vi "sgp4Init.vi"(1 "satrec":T2) -> (0 "satrec 2":T1)   [LabVIEW 2015]
uses:
  <vilib>/imath/engines/lvmath/Plug In/_Char/NIMS_CH_character datatype.ctl
  <vilib>/imath/engines/lvmath2/RunTimeEngine/Managers/WorkSpace/UID Generator.vi
  <vilib>/imath/engines/lvmath2/RunTimeEngine/RunTimeType/NIMS_RunTimeType_From StrictType (excl LVString).vi
  <instcachedir>/0/NIMS_RunTimeType_From StrictType (excl LVString)_EB1C38A9BC5048DA9ABDA8F781E54D21.lvgen/NIMS_RunTimeType_From StrictType (excl LVString)_EB1C38A9BC5048DA9ABDA8F781E54D21_032.vi
  <instcachedir>/0/NIMS_RunTimeType_From StrictType (excl LVString)_EB1C38A9BC5048DA9ABDA8F781E54D21.lvgen/NIMS_RunTimeType_From StrictType (excl LVString)_EB1C38A9BC5048DA9ABDA8F781E54D21_030.vi
  <vilib>/imath/engines/lvmath/Plug In/_Char/NIMS_CH_String CV to Character 2D.vi
  <instcachedir>/0/NIMS_CH_String CV to Character 2D_EC8CCB3F0D074D66A728E5B1D55F815A.lvgen/NIMS_CH_String CV to Character 2D_EC8CCB3F0D074D66A728E5B1D55F815A_000.vi
  <instcachedir>/0/NIMS_RunTimeType_From StrictType (excl LVString)_EB1C38A9BC5048DA9ABDA8F781E54D21.lvgen/NIMS_RunTimeType_From StrictType (excl LVString)_EB1C38A9BC5048DA9ABDA8F781E54D21_001.vi
  <instcachedir>/0/NIMS_RunTimeType_From StrictType (excl LVString)_EB1C38A9BC5048DA9ABDA8F781E54D21.lvgen/NIMS_RunTimeType_From StrictType (excl LVString)_EB1C38A9BC5048DA9ABDA8F781E54D21_031.vi
  <vilib>/imath/engines/lvmath2/RunTimeEngine/Struct/NIMS_StructSetField.vi
  <vilib>/imath/engines/lvmath2/RunTimeEngine/Struct/NIMS_StructGetField.vi
  <vilib>/imath/engines/lvmath2/RunTimeEngine/RunTimeType/NIMS_RunTimeType_To Numeric.vi
  <instcachedir>/0/NIMS_RunTimeType_To Numeric_B134FEC7BFC54ED5998F4CFD2EE98288.lvgen/NIMS_RunTimeType_To Numeric_B134FEC7BFC54ED5998F4CFD2EE98288_007.vi
  <instcachedir>/0/NIMS_RunTimeType_To Numeric_B134FEC7BFC54ED5998F4CFD2EE98288.lvgen/NIMS_RunTimeType_To Numeric_B134FEC7BFC54ED5998F4CFD2EE98288_009.vi
  <instcachedir>/0/NIMS_RunTimeType_From StrictType (excl LVString)_EB1C38A9BC5048DA9ABDA8F781E54D21.lvgen/NIMS_RunTimeType_From StrictType (excl LVString)_EB1C38A9BC5048DA9ABDA8F781E54D21_000.vi
  <vilib>/imath/engines/lvmath2/RunTimeEngine/LocalVariableDefStatement/MC_LocalVariableDefStatement_Display.vi
  <instcachedir>/0/NIMS_RunTimeType_To Numeric_B134FEC7BFC54ED5998F4CFD2EE98288.lvgen/NIMS_RunTimeType_To Numeric_B134FEC7BFC54ED5998F4CFD2EE98288_008.vi
  <vilib>/imath/engines/lvmath2/RunTimeEngine/BuiltInFunctions/cos/NIMS_cos(C).vi
  <instcachedir>/0/NIMS_cos(C)_840A8FDA839D4E2AADB43697F53F61ED.lvgen/NIMS_cos(C)_840A8FDA839D4E2AADB43697F53F61ED_001.vi
  <vilib>/imath/engines/lvmath2/RunTimeEngine/ArithmeticOperatorToken/NIMS_ArithmeticOperator_power(S).vi
  <instcachedir>/0/NIMS_ArithmeticOperator_power(S)_DFB67823F1414E5097C86E39787D8CA8.lvgen/NIMS_ArithmeticOperator_power(S)_DFB67823F1414E5097C86E39787D8CA8_009.vi
  <vilib>/imathl/engines/lvmath/Functions/Error Handling/Create Error.vi
  <vilib>/imath/engines/lvmath2/RunTimeEngine/BuiltInFunctions/sin/NIMS_sin(C).vi
  <instcachedir>/0/NIMS_sin(C)_93B37CF23FEA46B381CCAA607B2209DC.lvgen/NIMS_sin(C)_93B37CF23FEA46B381CCAA607B2209DC_001.vi
  <vilib>/imath/engines/lvmath2/RunTimeEngine/BuiltInFunctions/rem/NIMS_rem_no checks.vi
  <instcachedir>/0/NIMS_rem_no checks_948DC4F3B45040069021B8F54D02F312.lvgen/NIMS_rem_no checks_948DC4F3B45040069021B8F54D02F312_000.vi
  <vilib>/imath/engines/lvmath2/RunTimeEngine/BuiltInFunctions/abs/NIMS_abs(signed).vi
  <instcachedir>/0/NIMS_abs(signed)_C4FCB8E6058B49B797C7C8D53CA5F6EC.lvgen/NIMS_abs(signed)_C4FCB8E6058B49B797C7C8D53CA5F6EC_002.vi
  <instcachedir>/0/NIMS_ArithmeticOperator_power(S)_DFB67823F1414E5097C86E39787D8CA8.lvgen/NIMS_ArithmeticOperator_power(S)_DFB67823F1414E5097C86E39787D8CA8_014.vi
  <instcachedir>/0/NIMS_ArithmeticOperator_power(S)_DFB67823F1414E5097C86E39787D8CA8.lvgen/NIMS_ArithmeticOperator_power(S)_DFB67823F1414E5097C86E39787D8CA8_010.vi
  <vilib>/imath/engines/lvmath2/RunTimeEngine/BuiltInFunctions/atan2/NIMS_atan2.vi
  <instcachedir>/0/NIMS_atan2_A91AA4A7D42247EDBE8F76DB99AF04A4.lvgen/NIMS_atan2_A91AA4A7D42247EDBE8F76DB99AF04A4_000.vi
  <vilib>/imath/engines/lvmath2/RunTimeEngine/RangeToken/NIMS_Range_R2 - Integer.vi
  <instcachedir>/0/NIMS_Range_R2 - Integer_396D5D4FB869421F9245109A0975AD54.lvgen/NIMS_Range_R2 - Integer_396D5D4FB869421F9245109A0975AD54_000.vi
  <vilib>/imath/engines/lvmath2/RunTimeEngine/CommandStatement/MC_CommandStatement_break.vi
  <vilib>/imath/engines/lvmath2/RunTimeEngine/VariableToken/NIMS_VariableToken_CondDefined.vi
  <instcachedir>/0/NIMS_VariableToken_CondDefined_FE30D0A1BFB24F098D41DEBABFE96BE1.lvgen/NIMS_VariableToken_CondDefined_FE30D0A1BFB24F098D41DEBABFE96BE1_003.vi
  <vilib>/imath/engines/lvmath2/RunTimeEngine/ErrorHandling/NIMS_Create Error From Enums.vi
  <vilib>/imath/engines/lvmath/Plug In/_Char/RunTimeType/NIMS_CH_RunTimeType_To Character 2D.vi
  <vilib>/imath/engines/lvmath/Plug In/_Char/NIMS_CH_Character 2D to U8 2D.vi
  <vilib>/imath/engines/lvmath2/RunTimeSupport/NIMS_Complex To Real.vi
  <instcachedir>/0/NIMS_Complex To Real_01315F44AA8B4CE79FEF95AE999DC25E.lvgen/NIMS_Complex To Real_01315F44AA8B4CE79FEF95AE999DC25E_001.vi
  <instcachedir>/0/NIMS_abs(signed)_C4FCB8E6058B49B797C7C8D53CA5F6EC.lvgen/NIMS_abs(signed)_C4FCB8E6058B49B797C7C8D53CA5F6EC_000.vi
  <vilib>/imath/engines/lvmath/Plug In/_Char/NIMS_CH_Character 2D to String 1D.vi
  <vilib>/imath/engines/lvmath2/RunTimeEngine/Managers/SymbolTable/Clear UID.vi
  <vilib>/imath/engines/lvmath2/RunTimeEngine/NodeEndStatement/NIMS_NodeEndStatement_Output.vi
  <instcachedir>/0/NIMS_NodeEndStatement_Output_53EC0D466D134D7ABD903AC30B43404B.lvgen/NIMS_NodeEndStatement_Output_53EC0D466D134D7ABD903AC30B43404B_011.vi
  <vilib>/imath/engines/lvmath2/RunTimeEngine/ErrorHandling/NIMS_Finalize Error.vi
  <vilib>/imath/engines/lvmath2/RunTimeEngine/Managers/SymbolTable/NIMS_WorkSpace.lvlib
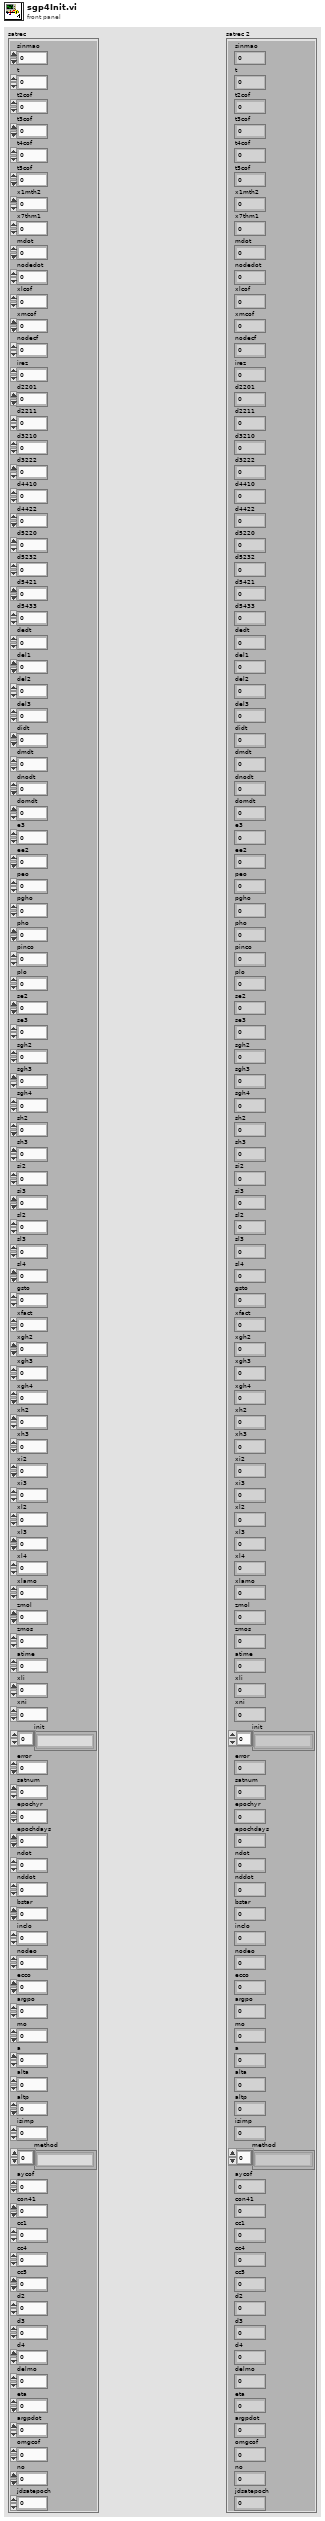
[diagram p1: front panel]
types:
  T1 = cluster{"sinmao":cdb, "t":dbl, "t2cof":cdb, "t3cof":cdb, "t4cof":cdb, "t5cof":cdb, "x1mth2":cdb, "x7thm1":cdb, "mdot":cdb, "nodedot":cdb, "xlcof":cdb, "xmcof":cdb, "nodecf":cdb, "irez":sgl, "d2201":dbl, "d2211":dbl, "d3210":dbl, "d3222":dbl, "d4410":dbl, "d4422":dbl, "d5220":dbl, "d5232":dbl, "d5421":dbl, "d5433":dbl, "dedt":dbl, "del1":dbl, "del2":dbl, "del3":dbl, "didt":dbl, "dmdt":dbl, "dnodt":dbl, "domdt":dbl, "e3":cdb, "ee2":cdb, "peo":dbl, "pgho":dbl, "pho":dbl, "pinco":dbl, "plo":dbl, "se2":cdb, "se3":cdb, "sgh2":cdb, "sgh3":cdb, "sgh4":cdb, "sh2":cdb, "sh3":cdb, "si2":cdb, "si3":cdb, "sl2":cdb, "sl3":cdb, "sl4":cdb, "gsto":dbl, "xfact":dbl, "xgh2":cdb, "xgh3":cdb, "xgh4":cdb, "xh2":cdb, "xh3":cdb, "xi2":cdb, "xi3":cdb, "xl2":cdb, "xl3":cdb, "xl4":cdb, "xlamo":dbl, "zmol":dbl, "zmos":dbl, "atime":dbl, "xli":dbl, "xni":dbl, "init":string[], "error":sgl, "satnum":sgl, "epochyr":sgl, "epochdays":dbl, "ndot":dbl, "nddot":dbl, "bstar":dbl, "inclo":cdb, "nodeo":cdb, "ecco":cdb, "argpo":cdb, "mo":cdb, "a":cdb, "alta":cdb, "altp":cdb, "isimp":sgl, "method":string[], "aycof":cdb, "con41":cdb, "cc1":cdb, "cc4":cdb, "cc5":cdb, "d2":cdb, "d3":cdb, "d4":cdb, "delmo":cdb, "eta":cdb, "argpdot":cdb, "omgcof":cdb, "no":cdb, "jdsatepoch":dbl}
  T2 = cluster{"sinmao":sgl, "t":sgl, "t2cof":sgl, "t3cof":sgl, "t4cof":sgl, "t5cof":sgl, "x1mth2":sgl, "x7thm1":sgl, "mdot":sgl, "nodedot":sgl, "xlcof":sgl, "xmcof":sgl, "nodecf":sgl, "irez":sgl, "d2201":sgl, "d2211":sgl, "d3210":sgl, "d3222":sgl, "d4410":sgl, "d4422":sgl, "d5220":sgl, "d5232":sgl, "d5421":sgl, "d5433":sgl, "dedt":sgl, "del1":sgl, "del2":sgl, "del3":sgl, "didt":sgl, "dmdt":sgl, "dnodt":sgl, "domdt":sgl, "e3":sgl, "ee2":sgl, "peo":sgl, "pgho":sgl, "pho":sgl, "pinco":sgl, "plo":sgl, "se2":sgl, "se3":sgl, "sgh2":sgl, "sgh3":sgl, "sgh4":sgl, "sh2":sgl, "sh3":sgl, "si2":sgl, "si3":sgl, "sl2":sgl, "sl3":sgl, "sl4":sgl, "gsto":sgl, "xfact":sgl, "xgh2":sgl, "xgh3":sgl, "xgh4":sgl, "xh2":sgl, "xh3":sgl, "xi2":sgl, "xi3":sgl, "xl2":sgl, "xl3":sgl, "xl4":sgl, "xlamo":sgl, "zmol":sgl, "zmos":sgl, "atime":sgl, "xli":sgl, "xni":sgl, "init":string[], "error":sgl, "satnum":sgl, "epochyr":sgl, "epochdays":dbl, "ndot":dbl, "nddot":dbl, "bstar":dbl, "inclo":dbl, "nodeo":dbl, "ecco":dbl, "argpo":dbl, "mo":dbl, "a":cdb, "alta":cdb, "altp":cdb, "isimp":sgl, "method":string[], "aycof":sgl, "con41":sgl, "cc1":sgl, "cc4":sgl, "cc5":sgl, "d2":sgl, "d3":sgl, "d4":sgl, "delmo":sgl, "eta":sgl, "argpdot":sgl, "omgcof":sgl, "no":dbl, "jdsatepoch":dbl}
  T3 = cluster{"sinmao":cdb, "t":dbl, "t2cof":cdb, "t3cof":cdb, "t4cof":cdb, "t5cof":cdb, "x1mth2":cdb, "x7thm1":cdb, "mdot":cdb, "nodedot":cdb, "xlcof":cdb, "xmcof":cdb, "nodecf":cdb, "irez":sgl, "d2201":cdb, "d2211":cdb, "d3210":cdb, "d3222":cdb, "d4410":cdb, "d4422":cdb, "d5220":cdb, "d5232":cdb, "d5421":cdb, "d5433":cdb, "dedt":cdb, "del1":cdb, "del2":cdb, "del3":cdb, "didt":cdb, "dmdt":cdb, "dnodt":cdb, "domdt":cdb, "e3":cdb, "ee2":cdb, "peo":dbl, "pgho":dbl, "pho":dbl, "pinco":dbl, "plo":dbl, "se2":cdb, "se3":cdb, "sgh2":cdb, "sgh3":cdb, "sgh4":cdb, "sh2":cdb, "sh3":cdb, "si2":cdb, "si3":cdb, "sl2":cdb, "sl3":cdb, "sl4":cdb, "gsto":dbl, "xfact":cdb, "xgh2":cdb, "xgh3":cdb, "xgh4":cdb, "xh2":cdb, "xh3":cdb, "xi2":cdb, "xi3":cdb, "xl2":cdb, "xl3":cdb, "xl4":cdb, "xlamo":dbl, "zmol":dbl, "zmos":dbl, "atime":dbl, "xli":dbl, "xni":cdb, "init":string[], "error":sgl, "satnum":sgl, "epochyr":sgl, "epochdays":dbl, "ndot":dbl, "nddot":dbl, "bstar":dbl, "inclo":cdb, "nodeo":cdb, "ecco":cdb, "argpo":cdb, "mo":cdb, "a":cdb, "alta":cdb, "altp":cdb, "isimp":sgl, "method":string[], "aycof":cdb, "con41":cdb, "cc1":cdb, "cc4":cdb, "cc5":cdb, "d2":cdb, "d3":cdb, "d4":cdb, "delmo":cdb, "eta":cdb, "argpdot":cdb, "omgcof":cdb, "no":cdb, "jdsatepoch":dbl}
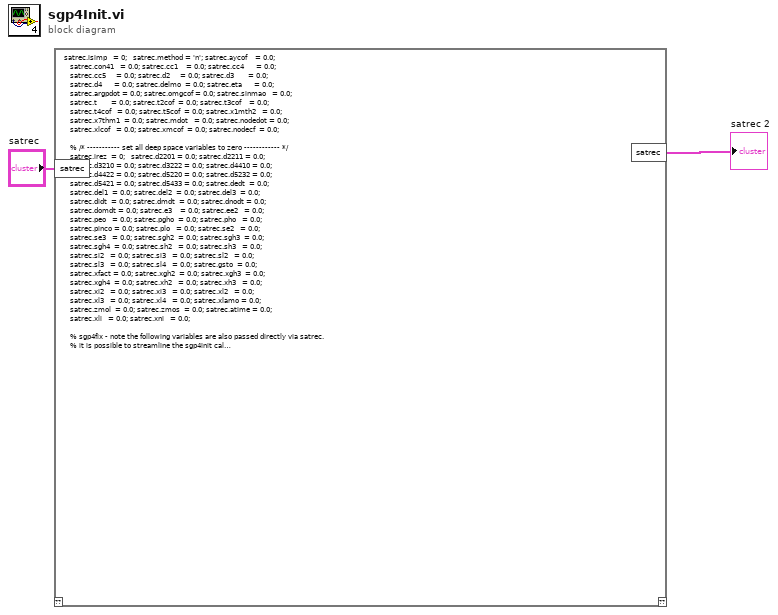
[diagram p0: block diagram]
diagram:
  n1 = mathscript code="satrec.isimp   = 0;   satrec.method = 'n'; satrec.aycof    = 0.0;\n   satrec.con41   = 0.0; satrec.cc1    = 0.0; satrec.cc4      = 0.0;\n   satrec.cc5     = 0.0; satrec.d2     = 0.0; satrec.d3       = 0.0;\n   satrec.d4      = 0.0; satrec.delmo  = 0.0; satrec.eta      = 0.0;\n   satrec.argpdot = 0.0; satrec.omgcof = 0.0; satrec.sinmao   = 0.0;\n   satrec.t       = 0.0; satrec.t2cof  = 0.0; satrec.t3cof    = 0.0;\n   satrec.t4cof   = 0.0; satrec.t5cof  = 0.0; satrec.x1mth2   = 0.0;\n   satrec.x7thm1  = 0.0; satrec.mdot   = 0.0; satrec.nodedot = 0.0;\n   satrec.xlcof   = 0.0; satrec.xmcof  = 0.0; satrec.nodecf  = 0.0;\n\n   % /* ----------- set all deep space variables to zero ------------ */\n   satrec.irez  = 0;   satrec.d2201 = 0.0; satrec.d2211 = 0.0;\n   satrec.d3210 = 0.0; satrec.d3222 = 0.0; satrec.d4410 = 0.0;\n   satrec.d4422 = 0.0; satrec.d5220 = 0.0; satrec.d5232 = 0.0;\n   satrec.d5421 = 0.0; satrec.d5433 = 0.0; satrec.dedt  = 0.0;\n   satrec.del1  = 0.0; satrec.del2  = 0.0; satrec.del3  = 0.0;\n   satrec.didt  = 0.0; satrec.dmdt  = 0.0; satrec.dnodt = 0.0;\n   satrec.domdt = 0.0; satrec.e3    = 0.0; satrec.ee2   = 0.0;\n   satrec.peo   = 0.0; satrec.pgho  = 0.0; satrec.pho   = 0.0;\n   satrec.pinco = 0.0; satrec.plo   = 0.0; satrec.se2   = 0.0;\n   satrec.se3   = 0.0; satrec.sgh2  = 0.0; satrec.sgh3  = 0.0;\n   satrec.sgh4  = 0.0; satrec.sh2   = 0.0; satrec.sh3   = 0.0;\n   satrec.si2   = 0.0; satrec.si3   = 0.0; satrec.sl2   = 0.0;\n   satrec.sl3   = 0.0; satrec.sl4   = 0.0; satrec.gsto  = 0.0;\n   satrec.xfact = 0.0; satrec.xgh2  = 0.0; satrec.xgh3  = 0.0;\n   satrec.xgh4  = 0.0; satrec.xh2   = 0.0; satrec.xh3   = 0.0;\n   satrec.xi2   = 0.0; satrec.xi3   = 0.0; satrec.xl2   = 0.0;\n   satrec.xl3   = 0.0; satrec.xl4   = 0.0; satrec.xlamo = 0.0;\n   satrec.zmol  = 0.0; satrec.zmos  = 0.0; satrec.atime = 0.0;\n   satrec.xli   = 0.0; satrec.xni   = 0.0;\n\n   % sgp4fix - note the following variables are also passed directly via satrec. \n   % it is possible to streamline the sgp4init call by deleting the \"x\"\n   % variables, but the user would need to set the satrec.* values first. we\n   % include the additional assignment in case twoline2rv is not used. \n   %satrec.bstar      = xbstar;\n   %satrec.ecco       = xecco;\n   %satrec.argpo      = xargpo;\n   %satrec.inclo      = xinclo;\n   %satrec.mo         = xmo;\n   %satrec.no         = xno;\n   %satrec.nodeo      = xnodeo;\n\n   %     /* -------------------- wgs-72 earth constants ----------------- */\n   %     // sgp4fix identify constants and allow alternate values\n   %global tumin mu radiusearthkm xke j2 j3 j4 j3oj2  \n  % [tumin, mu, radiusearthkm, xke, j2, j3, j4, j3oj2] = getgravc( whichconst );\n           mu     = 398600.79964;        %// in km3 / s2\n           radiusearthkm = 6378.135;     %// km\n           xke    = 0.0743669161;\n           tumin  = 1.0 / xke;\n           j2     =   0.001082616;\n           j3     =  -0.00000253881;\n           j4     =  -0.00000165597;\n           j3oj2  =  j3 / j2;\n\n\n   ss     = 78.0 / radiusearthkm + 1.0;\n   qzms2t = ((120.0 - 78.0) / radiusearthkm)^4;\n   x2o3   =  2.0 / 3.0;\n   % // sgp4fix divisor for divide by zero check on inclination\n   temp4  =   1.0 + cos(pi-1.0e-9);\n\n   satrec.init = 'y';\n   satrec.t    = 0.0;\n\n % [ainv,  ao,     satrec.con41,   con42,  cosio,  cosio2, einv,   eccsq,...\n  %         satrec.method,  omeosq, posq,   rp,     rteosq, sinio,...\n   %      satrec.gsto,    satrec.no] = initl(satrec.ecco,    satrec.jdsatepoch,  satrec.inclo,   satrec.no,...\n     %     satrec.satnum);\n\n%------------ Function initl.m --------------------------------------------------\necco = satrec.ecco;\nepoch = satrec.jdsatepoch;\ninclo =  satrec.inclo,\nno= satrec.no;\nsatn = satrec.satnum;\n\n x2o3   = 2.0 / 3.0;\n\n   % /* ------------- calculate auxillary epoch quantities ---------- */\n   eccsq  = ecco * ecco;\n   omeosq = 1.0 - eccsq;\n   rteosq = sqrt(omeosq);\n   cosio  = cos(inclo);\n   cosio2 = cosio * cosio;\n\n   % /* ------------------ un-kozai the mean motion ----------------- */\n   ak    = (xke / no)^x2o3;\n   d1    = 0.75 * j2 * (3.0 * cosio2 - 1.0) / (rteosq * omeosq);\n   del   = d1 / (ak * ak);\n   adel  = ak * (1.0 - del * del - del *...\n       (1.0 / 3.0 + 134.0 * del * del / 81.0));\n   del   = d1/(adel * adel);\n   no    = no / (1.0 + del);\n\n   ao    = (xke / no)^x2o3;\n   sinio = sin(inclo);\n   po    = ao * omeosq;\n   con42 = 1.0 - 5.0 * cosio2;\n   con41 = -con42-cosio2-cosio2;\n   ainv  = 1.0 / ao;\n   einv  = 1.0 / ecco;\n   posq  = po * po;\n   rp    = ao * (1.0 - ecco);\n   method = 'n';\n\n   % sgp4fix modern approach to finding sidereal time\n   % gsto = gstime(epoch + 2433281.5);\n\n   % sgp4fix use old way of finding gst\n   % count integer number of days from 0 jan 1970\n   ts70  = epoch - 7305.0;\n   ids70 = floor(ts70 + 1.0e-8);\n   ds70  = ids70;\n   tfrac = ts70 - ds70;\n   % find greenwich location at epoch\n   c1    = 1.72027916940703639e-2;\n   thgr70= 1.7321343856509374;\n   fk5r  = 5.07551419432269442e-15;\n   twopi = 6.283185307179586;\n   c1p2p = c1 + twopi;\n   gsto  = rem( thgr70 + c1*ds70 + c1p2p*tfrac + ts70*ts70*fk5r, twopi);\n   if ( gsto < 0.0 )\n       gsto = gsto + twopi;\n   end;\n\nsatrec.con41 = con41;\nsatrec.method = method;\nsatrec.gsto = gsto;\nsatrec.no = no;\n%-------------------------------------------------------------------------\n\n satrec.error = 0;\n       \n   if (rp < 1.0)\n   %   printf(\"# *** satn%d epoch elts sub-orbital ***\\n\", satn);\n       satrec.error = 5;\n   end\n\n   if ((omeosq >= 0.0 ) | ( satrec.no >= 0.0))\n       satrec.isimp = 0;\n       if (rp < (220.0 / radiusearthkm + 1.0))\n           satrec.isimp = 1;\n       end\n       sfour  = ss;\n       qzms24 = qzms2t;\n       perige = (rp - 1.0) * radiusearthkm;\n\n       % /* - for perigees below 156 km, s and qoms2t are altered - */\n       if (perige < 156.0)\n           sfour = perige - 78.0;\n           if (perige < 98.0)\n               sfour = 20.0;\n           end\n           qzms24 = ((120.0 - sfour) / radiusearthkm)^4.0;\n           sfour  = sfour / radiusearthkm + 1.0;\n       end\n       pinvsq = 1.0 / posq;\n\n       tsi  = 1.0 / (ao - sfour);\n       satrec.eta  = ao * satrec.ecco * tsi;\n       etasq = satrec.eta * satrec.eta;\n       eeta  = satrec.ecco * satrec.eta;\n       psisq = abs(1.0 - etasq);\n       coef  = qzms24 * tsi^4.0;\n       coef1 = coef / psisq^3.5;\n       cc2   = coef1 * satrec.no * (ao * (1.0 + 1.5 * etasq + eeta *...\n           (4.0 + etasq)) + 0.375 * j2 * tsi / psisq * satrec.con41 *...\n           (8.0 + 3.0 * etasq * (8.0 + etasq)));\n       satrec.cc1   = satrec.bstar * cc2;\n       cc3   = 0.0;\n       if (satrec.ecco > 1.0e-4)\n           cc3 = -2.0 * coef * tsi * j3oj2 * satrec.no * sinio / satrec.ecco;\n       end\n       satrec.x1mth2 = 1.0 - cosio2;\n       satrec.cc4    = 2.0* satrec.no * coef1 * ao * omeosq *...\n           (satrec.eta * (2.0 + 0.5 * etasq) + satrec.ecco *...\n           (0.5 + 2.0 * etasq) - j2 * tsi / (ao * psisq) *...\n           (-3.0 * satrec.con41 * (1.0 - 2.0 * eeta + etasq *...\n           (1.5 - 0.5 * eeta)) + 0.75 * satrec.x1mth2 *...\n           (2.0 * etasq - eeta * (1.0 + etasq)) * cos(2.0 * satrec.argpo)));\n       satrec.cc5 = 2.0 * coef1 * ao * omeosq * (1.0 + 2.75 *...\n           (etasq + eeta) + eeta * etasq);\n       cosio4 = cosio2 * cosio2;\n       temp1  = 1.5 * j2 * pinvsq * satrec.no;\n       temp2  = 0.5 * temp1 * j2 * pinvsq;\n       temp3  = -0.46875 * j4 * pinvsq * pinvsq * satrec.no;\n       satrec.mdot     = satrec.no + 0.5 * temp1 * rteosq * satrec.con41 +...\n           0.0625 * temp2 * rteosq * (13.0 - 78.0 * cosio2 + 137.0 * cosio4);\n       satrec.argpdot  = -0.5 * temp1 * con42 + 0.0625 * temp2 *...\n           (7.0 - 114.0 * cosio2 + 395.0 * cosio4) +...\n           temp3 * (3.0 - 36.0 * cosio2 + 49.0 * cosio4);\n       xhdot1            = -temp1 * cosio;\n       satrec.nodedot = xhdot1 + (0.5 * temp2 * (4.0 - 19.0 * cosio2) +...\n           2.0 * temp3 * (3.0 - 7.0 * cosio2)) * cosio;\n       xpidot            =  satrec.argpdot+ satrec.nodedot;\n       satrec.omgcof   = satrec.bstar * cc3 * cos(satrec.argpo);\n       satrec.xmcof    = 0.0;\n       if (satrec.ecco > 1.0e-4)\n           satrec.xmcof = -x2o3 * coef * satrec.bstar / eeta;\n       end\n       satrec.nodecf = 3.5 * omeosq * xhdot1 * satrec.cc1;\n       satrec.t2cof   = 1.5 * satrec.cc1;\n\n       % // sgp4fix for divide by zero with xinco = 180 deg\n       if (abs(cosio+1.0) > 1.5e-12)\n          satrec.xlcof   = -0.25 * j3oj2 * sinio *...\n              (3.0 + 5.0 * cosio) / (1.0 + cosio);\n       else\n         satrec.xlcof   = -0.25 * j3oj2 * sinio *...\n              (3.0 + 5.0 * cosio) / temp4;\n       end   \n       satrec.aycof   = -0.5 * j3oj2 * sinio;\n       satrec.delmo   = (1.0 + satrec.eta * cos(satrec.mo))^3;\n       satrec.sinmao  = sin(satrec.mo);\n       satrec.x7thm1  = 7.0 * cosio2 - 1.0;\n\n       % /* --------------- deep space initialization ------------- */\n       if ((2*pi / satrec.no) >= 225.0)\n           satrec.method = 'd';\n           satrec.isimp  = 1;\n           tc    =  0.0;\n           inclm = satrec.inclo;\n\n   %        [sinim,cosim,sinomm,cosomm,snodm,cnodm,day,satrec.e3,satrec.ee2,...\n    %           em,emsq,gam,satrec.peo,satrec.pgho,satrec.pho,satrec.pinco,...\n     %          satrec.plo,rtemsq,satrec.se2,satrec.se3,satrec.sgh2,...\n      %         satrec.sgh3,satrec.sgh4,satrec.sh2,satrec.sh3,satrec.si2,...\n      %         satrec.si3,satrec.sl2,satrec.sl3,satrec.sl4,s1,s2,s3,s4,s5,...\n      %         s6,s7,ss1,ss2,ss3,ss4,ss5,ss6,ss7,sz1,sz2,sz3,sz11,sz12,...\n      %         sz13,sz21,sz22,sz23,sz31,sz32,sz33,satrec.xgh2,satrec.xgh3,...\n       %        satrec.xgh4,satrec.xh2,satrec.xh3,satrec.xi2,satrec.xi3,...\n       %       satrec.xl2,satrec.xl3,satrec.xl4,nm,z1,z2,z3,z11,z12,z13,...\n       %       z21,z22,z23,z31,z32,z33,satrec.zmol,satrec.zmos] = ...\n      %       dscom(satrec.jdsatepoch,satrec.ecco,satrec.argpo,tc,satrec.inclo,...\n       %       satrec.nodeo,satrec.no);\n\n%---------------------function dscom-----------------------------\n\nepoch = satrec.jdsatepoch;\nep = satrec.ecco;\nargpp = satrec.argpo;\ninclp = satrec.inclo;\nnodep = satrec.nodeo;\nnp = satrec.no;\n\n  % /* -------------------------- constants ------------------------- */\n   zes     =  0.01675;\n   zel     =  0.05490;\n   c1ss    =  2.9864797e-6;\n   c1l     =  4.7968065e-7;\n   zsinis  =  0.39785416;\n   zcosis  =  0.91744867;\n   zcosgs  =  0.1945905;\n   zsings  = -0.98088458;\n   twopi   =  2.0 * pi;\n\n   % /* --------------------- local variables ------------------------ */\n   nm     = np;\n   em     = ep;\n   snodm  = sin(nodep);\n   cnodm  = cos(nodep);\n   sinomm = sin(argpp);\n   cosomm = cos(argpp);\n   sinim  = sin(inclp);\n   cosim  = cos(inclp);\n   emsq   = em * em;\n   betasq = 1.0 - emsq;\n   rtemsq = sqrt(betasq);\n\n   % /* ----------------- initialize lunar solar terms --------------- */\n   peo    = 0.0;\n   pinco  = 0.0;\n   plo    = 0.0;\n   pgho   = 0.0;\n   pho    = 0.0;\n   day    = epoch + 18261.5 + tc / 1440.0;\n   xnodce = rem(4.5236020 - 9.2422029e-4 * day, twopi);\n   stem   = sin(xnodce);\n   ctem   = cos(xnodce);\n   zcosil = 0.91375164 - 0.03568096 * ctem;\n   zsinil = sqrt(1.0 - zcosil * zcosil);\n   zsinhl = 0.089683511 * stem / zsinil;\n   zcoshl = sqrt(1.0 - zsinhl * zsinhl);\n   gam    = 5.8351514 + 0.0019443680 * day;\n   zx     = 0.39785416 * stem / zsinil;\n   zy     = zcoshl * ctem + 0.91744867 * zsinhl * stem;\n   zx     = atan2(zx, zy);\n   zx     = gam + zx - xnodce;\n   zcosgl = cos(zx);\n   zsingl = sin(zx);\n\n   % /* ------------------------- do solar terms --------------------- */\n   zcosg = zcosgs;\n   zsing = zsings;\n   zcosi = zcosis;\n   zsini = zsinis;\n   zcosh = cnodm;\n   zsinh = snodm;\n   cc    = c1ss;\n   xnoi  = 1.0 / nm;\n\n   for (lsflg = 1:2)\n       a1  =   zcosg * zcosh + zsing * zcosi * zsinh;\n       a3  =  -zsing * zcosh + zcosg * zcosi * zsinh;\n       a7  =  -zcosg * zsinh + zsing * zcosi * zcosh;\n       a8  =   zsing * zsini;\n       a9  =   zsing * zsinh + zcosg * zcosi * zcosh;\n       a10 =   zcosg * zsini;\n       a2  =   cosim * a7 + sinim * a8;\n       a4  =   cosim * a9 + sinim * a10;\n       a5  =  -sinim * a7 + cosim * a8;\n       a6  =  -sinim * a9 + cosim * a10;\n\n       x1  =  a1 * cosomm + a2 * sinomm;\n       x2  =  a3 * cosomm + a4 * sinomm;\n       x3  = -a1 * sinomm + a2 * cosomm;\n       x4  = -a3 * sinomm + a4 * cosomm;\n       x5  =  a5 * sinomm;\n       x6  =  a6 * sinomm;\n       x7  =  a5 * cosomm;\n       x8  =  a6 * cosomm;\n\n       z31 = 12.0 * x1 * x1 - 3.0 * x3 * x3;\n       z32 = 24.0 * x1 * x2 - 6.0 * x3 * x4;\n       z33 = 12.0 * x2 * x2 - 3.0 * x4 * x4;\n       z1  =  3.0 *  (a1 * a1 + a2 * a2) + z31 * emsq;\n       z2  =  6.0 *  (a1 * a3 + a2 * a4) + z32 * emsq;\n       z3  =  3.0 *  (a3 * a3 + a4 * a4) + z33 * emsq;\n       z11 = -6.0 * a1 * a5 + emsq *  (-24.0 * x1 * x7-6.0 * x3 * x5);\n       z12 = -6.0 *  (a1 * a6 + a3 * a5) + emsq *...\n           (-24.0 * (x2 * x7 + x1 * x8) - 6.0 * (x3 * x6 + x4 * x5));\n       z13 = -6.0 * a3 * a6 + emsq * (-24.0 * x2 * x8 - 6.0 * x4 * x6);\n       z21 =  6.0 * a2 * a5 + emsq * (24.0 * x1 * x5 - 6.0 * x3 * x7);\n       z22 =  6.0 *  (a4 * a5 + a2 * a6) + emsq *...\n           (24.0 * (x2 * x5 + x1 * x6) - 6.0 * (x4 * x7 + x3 * x8));\n       z23 =  6.0 * a4 * a6 + emsq * (24.0 * x2 * x6 - 6.0 * x4 * x8);\n       z1  = z1 + z1 + betasq * z31;\n       z2  = z2 + z2 + betasq * z32;\n       z3  = z3 + z3 + betasq * z33;\n       s3  = cc * xnoi;\n       s2  = -0.5 * s3 / rtemsq;\n       s4  = s3 * rtemsq;\n       s1  = -15.0 * em * s4;\n       s5  = x1 * x3 + x2 * x4;\n       s6  = x2 * x3 + x1 * x4;\n       s7  = x2 * x4 - x1 * x3;\n\n       % /* ----------------------- do lunar terms ------------------- */\n       if (lsflg == 1)\n           ss1   = s1;\n           ss2   = s2;\n           ss3   = s3;\n           ss4   = s4;\n           ss5   = s5;\n           ss6   = s6;\n           ss7   = s7;\n           sz1   = z1;\n           sz2   = z2;\n           sz3   = z3;\n           sz11  = z11;\n           sz12  = z12;\n           sz13  = z13;\n           sz21  = z21;\n           sz22  = z22;\n           sz23  = z23;\n           sz31  = z31;\n           sz32  = z32;\n           sz33  = z33;\n           zcosg = zcosgl;\n           zsing = zsingl;\n           zcosi = zcosil;\n           zsini = zsinil;\n           zcosh = zcoshl * cnodm + zsinhl * snodm;\n           zsinh = snodm * zcoshl - cnodm * zsinhl;\n           cc    = c1l;\n       end\n   end\n\n   zmol = rem(4.7199672 + 0.22997150  * day - gam, twopi);\n   zmos = rem(6.2565837 + 0.017201977 * day, twopi);\n\n   % /* ------------------------ do solar terms ---------------------- */\n   se2  =   2.0 * ss1 * ss6;\n   se3  =   2.0 * ss1 * ss7;\n   si2  =   2.0 * ss2 * sz12;\n   si3  =   2.0 * ss2 * (sz13 - sz11);\n   sl2  =  -2.0 * ss3 * sz2;\n   sl3  =  -2.0 * ss3 * (sz3 - sz1);\n   sl4  =  -2.0 * ss3 * (-21.0 - 9.0 * emsq) * zes;\n   sgh2 =   2.0 * ss4 * sz32;\n   sgh3 =   2.0 * ss4 * (sz33 - sz31);\n   sgh4 = -18.0 * ss4 * zes;\n   sh2  =  -2.0 * ss2 * sz22;\n   sh3  =  -2.0 * ss2 * (sz23 - sz21);\n\n   % /* ------------------------ do lunar terms ---------------------- */\n   ee2  =   2.0 * s1 * s6;\n   e3   =   2.0 * s1 * s7;\n   xi2  =   2.0 * s2 * z12;\n   xi3  =   2.0 * s2 * (z13 - z11);\n   xl2  =  -2.0 * s3 * z2;\n   xl3  =  -2.0 * s3 * (z3 - z1);\n   xl4  =  -2.0 * s3 * (-21.0 - 9.0 * emsq) * zel;\n   xgh2 =   2.0 * s4 * z32;\n   xgh3 =   2.0 * s4 * (z33 - z31);\n   xgh4 = -18.0 * s4 * zel;\n   xh2  =  -2.0 * s2 * z22;\n   xh3  =  -2.0 * s2 * (z23 - z21);\n\nsatrec.e3  = e3;\nsatrec.ee2 = ee2;\nsatrec.peo = peo;\n satrec.pgho = pgho;\nsatrec.pho = pho;\n satrec.pinco = pinco;\n satrec.plo = plo;\n satrec.se2 = se2;\n satrec.se3 = se3;\nsatrec.sgh2 = sgh2;\nsatrec.sgh3 = sgh3;\nsatrec.sgh4 = sgh4;\nsatrec.sh2 = sh2;\nsatrec.sh3 = sh3;\nsatrec.si2 = si2;\nsatrec.si3 = si3;\n satrec.sl2 = sl2;\nsatrec.sl3 = sl3;\n satrec.sl4 = sl4;\n satrec.xgh2 = xgh2;\n satrec.xgh3 = xgh3;\n satrec.xgh4 = xgh4;\nsatrec.xh2 = xh2;\nsatrec.xh3 = xh3;\nsatrec.xi2 = xi2;\nsatrec.xi3 = xi3;\nsatrec.xl2 = xl2;\nsatrec.xl3 = xl3;\nsatrec.xl4 = xl4;\nsatrec.zmol = zmol;\nsatrec.zmos = zmos;\n\n%-------------------------------end function dscom----------------------------------------------\n% ---------- dpper-------------------------------------\n\n         %  [satrec.ecco,satrec.inclo,satrec.nodeo,satrec.argpo,satrec.mo]...\n          %     = dpper(satrec.e3,satrec.ee2,satrec.peo,satrec.pgho,...\n            %   satrec.pho,satrec.pinco,satrec.plo,satrec.se2,satrec.se3,...\n           %    satrec.sgh2,satrec.sgh3,satrec.sgh4,satrec.sh2,satrec.sh3,...\n          %     satrec.si2,satrec.si3,satrec.sl2,satrec.sl3,satrec.sl4,...\n            %   satrec.t,satrec.xgh2,satrec.xgh3,satrec.xgh4,satrec.xh2,...\n       %        satrec.xh3,satrec.xi2,satrec.xi3,satrec.xl2,satrec.xl3,...\n           %    satrec.xl4,satrec.zmol,satrec.zmos,inclm,satrec.init,...\n          %     satrec.ecco,satrec.inclo,satrec.nodeo,satrec.argpo,satrec.mo);\n\ne3 = satrec.e3;\nee2 = satrec.ee2;\npeo = satrec.peo;\npgho = satrec.pgho;\npho =  satrec.pho;\npinco = satrec.pinco;\nplo = satrec.plo;\nse2 = satrec.se2;\nse3 = satrec.se3;\nsgh2 = satrec.sgh2;\nsgh3 = satrec.sgh3;\nsgh4=satrec.sgh4;\nsh2 = satrec.sh2;\nsh3 =satrec.sh3;\nsi2 = satrec.si2;\nsi3 = satrec.si3;\nsl2 = satrec.sl2;\nsl3 = satrec.sl3;\nsl4 = satrec.sl4;\nt = satrec.t;\nxgh2 = satrec.xgh2;\nxgh3 = satrec.xgh3;\nxgh4 = satrec.xgh4;\nxh2 = satrec.xh2;\nxh3= satrec.xh3;\nxi2 = satrec.xi2;\nxi3 = satrec.xi3;\nxl2 = satrec.xl2;\nxl3 = satrec.xl3; \nxl4 = satrec.xl4;\nzmol = satrec.zmol;\nzmos = satrec.zmos;\ninit = satrec.init;\nep = satrec.ecco;\ninclo = satrec.inclo;\nnodep = satrec.nodeo;\nargpp = satrec.argpo;\nmp = satrec.mo;\n\n\n% /* --------------------- local variables ------------------------ */\n   twopi = 2.0 * pi;\n\n   % /* ---------------------- constants ----------------------------- */\n   zns   = 1.19459e-5;\n   zes   = 0.01675;\n   znl   = 1.5835218e-4;\n   zel   = 0.05490;\n\n   % /* --------------- calculate time varying periodics ----------- */\n   zm    = zmos + zns * t;\n   % // be sure that the initial call has time set to zero\n   if (init == 'y')\n       zm = zmos;\n   end\n   zf    = zm + 2.0 * zes * sin(zm);\n   sinzf = sin(zf);\n   f2    =  0.5 * sinzf * sinzf - 0.25;\n   f3    = -0.5 * sinzf * cos(zf);\n   ses   = se2* f2 + se3 * f3;\n   sis   = si2 * f2 + si3 * f3;\n   sls   = sl2 * f2 + sl3 * f3 + sl4 * sinzf;\n   sghs  = sgh2 * f2 + sgh3 * f3 + sgh4 * sinzf;\n   shs   = sh2 * f2 + sh3 * f3;\n   zm    = zmol + znl * t;\n   if (init == 'y')\n       zm = zmol;\n   end\n   zf    = zm + 2.0 * zel * sin(zm);\n   sinzf = sin(zf);\n   f2    =  0.5 * sinzf * sinzf - 0.25;\n   f3    = -0.5 * sinzf * cos(zf);\n   sel   = ee2 * f2 + e3 * f3;\n   sil   = xi2 * f2 + xi3 * f3;\n   sll   = xl2 * f2 + xl3 * f3 + xl4 * sinzf;\n   sghl  = xgh2 * f2 + xgh3 * f3 + xgh4 * sinzf;\n   shll  = xh2 * f2 + xh3 * f3;\n   pe    = ses + sel;\n   pinc  = sis + sil;\n   pl    = sls + sll;\n   pgh   = sghs + sghl;\n   ph    = shs + shll;\n\n   if (init == 'n')\n       %   //  0.2 rad = 11.45916 deg\n       pe    = pe - peo;\n       pinc  = pinc - pinco;\n       pl    = pl - plo;\n       pgh   = pgh - pgho;\n       ph    = ph - pho;\n       inclp = inclp + pinc;\n       ep    = ep + pe;\n       sinip = sin(inclp);\n       cosip = cos(inclp);\n\n       % /* ----------------- apply periodics directly ------------ */\n       %   //  sgp4fix for lyddane choice\n       %   //  strn3 used original inclination - this is technically feasible\n       %   //  gsfc used perturbed inclination - also technically feasible\n       %   //  probably best to readjust the 0.2 limit value and limit discontinuity\n       %   //  use next line for original strn3 approach and original inclination\n       %   //  if (inclo >= 0.2)\n       %   //  use next line for gsfc version and perturbed inclination\n       if (inclp >= 0.2)\n           ph     = ph / sinip;\n           pgh    = pgh - cosip * ph;\n           argpp  = argpp + pgh;\n           nodep  = nodep + ph;\n           mp     = mp + pl;\n       else\n           % /* ---- apply periodics with lyddane modification ---- */\n           sinop  = sin(nodep);\n           cosop  = cos(nodep);\n           alfdp  = sinip * sinop;\n           betdp  = sinip * cosop;\n           dalf   =  ph * cosop + pinc * cosip * sinop;\n           dbet   = -ph * sinop + pinc * cosip * cosop;\n           alfdp  = alfdp + dalf;\n           betdp  = betdp + dbet;\n           nodep  = rem(nodep, twopi);\n           % sgp4fix for afspc written intrinsic functions \n           % nodep used without a trigonometric function ahead \n           if (nodep < 0.0)\n               nodep = nodep + twopi;\n             end;\n           xls    = mp + argpp + cosip * nodep;\n           dls    = pl + pgh - pinc * nodep * sinip;\n           xls    = xls + dls;\n           xnoh   = nodep;\n           nodep  = atan2(alfdp, betdp);\n           % sgp4fix for afspc written intrinsic functions \n           % nodep used without a trigonometric function ahead \n           if (nodep < 0.0)\n               nodep = nodep + twopi;\n             end;\n           if (abs(xnoh - nodep) > pi)\n               if (nodep < xnoh)\n                   nodep = nodep + twopi;\n               else\n                   nodep = nodep - twopi;\n               end\n           end\n           mp    = mp + pl;\n           argpp = xls - mp - cosip * nodep;\n       end\n   end % // if init == 'n'\n\nsatrec.ecco = ep;\nsatrec.inclo = inclp;\nsatrec.nodeo = nodep;\nsatrec.argpo = argpp;\nsatrec.mo = mp;\n\n%--------------------end dpper.m------------------------------------------\n\n           argpm  = 0.0;\n           nodem  = 0.0;\n           mm     = 0.0;\n\n%-----------------begin dsinit.m -------------------------\nargpo = satrec.argpo;\nt=satrec.t;\ngsto=satrec.gsto;\nmo = satrec.mo;\nmdot = satrec.mdot;\nno =satrec.no;\nnodeo = satrec.nodeo;\nnodedot =satrec.nodedot\necco = satrec.ecco;\n\n % /* --------------------- local variables ------------------------ */\n   twopi = 2.0 * pi;\n   aonv  = 0.0;\n   q22    = 1.7891679e-6;\n   q31    = 2.1460748e-6;\n   q33    = 2.2123015e-7;\n   root22 = 1.7891679e-6;\n   root44 = 7.3636953e-9;\n   root54 = 2.1765803e-9;\n   rptim  = 4.37526908801129966e-3;\n   root32 = 3.7393792e-7;\n   root52 = 1.1428639e-7;\n   x2o3   = 2.0 / 3.0;\n   znl    = 1.5835218e-4;\n   zns    = 1.19459e-5;\n\n   %     // sgp4fix identify constants and allow alternate values\n   %global tumin mu radiusearthkm xke j2 j3 j4 j3oj2  \n\n   % /* -------------------- deep space initialization ------------ */\n   irez = 0;\n   if ((nm < 0.0052359877) && (nm > 0.0034906585))\n       irez = 1;\n   end\n   if ((nm >= 8.26e-3) && (nm <= 9.24e-3) && (em >= 0.5))\n       irez = 2;\n   end\n   d2201 = 0;\n   d2211 = 0;\n   d3210 = 0;\n   d3222 = 0;\n   d4410 = 0;\n   d4422 = 0;\n   d5220 = 0;\n   d5232 = 0;\n   d5421 = 0;\n   d5433 = 0;\n   del1  = 0;\n   del2  = 0;\n   del3  = 0;\n   atime = 0;\n   xfact = 0;\n   xlamo = 0;\n   xli   = 0;\n   xni   = 0;\n\n   % /* ------------------------ do solar terms ------------------- */\n   ses  =  ss1 * zns * ss5;\n   sis  =  ss2 * zns * (sz11 + sz13);\n   sls  = -zns * ss3 * (sz1 + sz3 - 14.0 - 6.0 * emsq);\n   sghs =  ss4 * zns * (sz31 + sz33 - 6.0);\n   shs  = -zns * ss2 * (sz21 + sz23);\n   %   // sgp4fix for 180 deg incl\n   if ((inclm < 5.2359877e-2) | (inclm > pi - 5.2359877e-2))\n       shs = 0.0;\n   end\n   if (sinim ~= 0.0)\n       shs = shs / sinim;\n   end\n   sgs  = sghs - cosim * shs;\n\n   % /* ------------------------- do lunar terms ------------------ */\n   dedt = ses + s1 * znl * s5;\n   didt = sis + s2 * znl * (z11 + z13);\n   dmdt = sls - znl * s3 * (z1 + z3 - 14.0 - 6.0 * emsq);\n   sghl = s4 * znl * (z31 + z33 - 6.0);\n   shll = -znl * s2 * (z21 + z23);\n   %   // sgp4fix for 180 deg incl\n   if ((inclm < 5.2359877e-2) | (inclm > pi - 5.2359877e-2))\n       shll = 0.0;\n   end\n   domdt = sgs + sghl;\n   dnodt = shs;\n   if (sinim ~= 0.0)\n       domdt = domdt - cosim / sinim * shll;\n       dnodt = dnodt + shll / sinim;\n   end\n\n   % /* ----------- calculate deep space resonance effects -------- */\n   dndt   = 0.0;\n   theta  = rem(gsto + tc * rptim, twopi);\n   em     = em + dedt * t;\n   inclm  = inclm + didt * t;\n   argpm  = argpm + domdt * t;\n   nodem  = nodem + dnodt * t;\n   mm     = mm + dmdt * t;\n   % //   sgp4fix for negative inclinations\n   % //   the following if statement should be commented out\n   % //if (inclm < 0.0)\n   % //  {\n   % //    inclm  = -inclm;\n   % //    argpm  = argpm - pi;\n   % //    nodem = nodem + pi;\n   % //  }\n\n   %  /* - update resonances : numerical (euler-maclaurin) integration - */\n   %  /* ------------------------- epoch restart ----------------------  */\n   %  //   sgp4fix for propagator problems\n   %  //   the following integration works for negative time steps and periods\n   %  //   the specific changes are unknown because the original code was so convoluted\n\n   % /* -------------- initialize the resonance terms ------------- */\n   if (irez ~= 0)\n       aonv = (nm / xke)^x2o3;\n\n       % /* ---------- geopotential resonance for 12 hour orbits ------ */\n       if (irez == 2)\n           cosisq = cosim * cosim;\n           emo    = em;\n           em     = ecco;\n           emsqo  = emsq;\n           emsq   = eccsq;\n           eoc    = em * emsq;\n           g201   = -0.306 - (em - 0.64) * 0.440;\n\n           if (em <= 0.65)\n               g211 =    3.616  -  13.2470 * em +  16.2900 * emsq;\n               g310 =  -19.302  + 117.3900 * em - 228.4190 * emsq +  156.5910 * eoc;\n               g322 =  -18.9068 + 109.7927 * em - 214.6334 * emsq +  146.5816 * eoc;\n               g410 =  -41.122  + 242.6940 * em - 471.0940 * emsq +  313.9530 * eoc;\n               g422 = -146.407  + 841.8800 * em - 1629.014 * emsq + 1083.4350 * eoc;\n               g520 = -532.114  + 3017.977 * em - 5740.032 * emsq + 3708.2760 * eoc;\n           else\n               g211 =   -72.099 +   331.819 * em -   508.738 * emsq +   266.724 * eoc;\n               g310 =  -346.844 +  1582.851 * em -  2415.925 * emsq +  1246.113 * eoc;\n               g322 =  -342.585 +  1554.908 * em -  2366.899 * emsq +  1215.972 * eoc;\n               g410 = -1052.797 +  4758.686 * em -  7193.992 * emsq +  3651.957 * eoc;\n               g422 = -3581.690 + 16178.110 * em - 24462.770 * emsq + 12422.520 * eoc;\n               if (em > 0.715)\n                   g520 =-5149.66 + 29936.92 * em - 54087.36 * emsq + 31324.56 * eoc;\n               else\n                   g520 = 1464.74 -  4664.75 * em +  3763.64 * emsq;\n               end\n           end\n           if (em < 0.7)\n               g533 = -919.22770 + 4988.6100 * em - 9064.7700 * emsq + 5542.21  * eoc;\n               g521 = -822.71072 + 4568.6173 * em - 8491.4146 * emsq + 5337.524 * eoc;\n               g532 = -853.66600 + 4690.2500 * em - 8624.7700 * emsq + 5341.4  * eoc;\n           else\n               g533 =-37995.780 + 161616.52 * em - 229838.20 * emsq + 109377.94 * eoc;\n               g521 =-51752.104 + 218913.95 * em - 309468.16 * emsq + 146349.42 * eoc;\n               g532 =-40023.880 + 170470.89 * em - 242699.48 * emsq + 115605.82 * eoc;\n           end\n\n           sini2=  sinim * sinim;\n           f220 =  0.75 * (1.0 + 2.0 * cosim+cosisq);\n           f221 =  1.5 * sini2;\n           f321 =  1.875 * sinim  *  (1.0 - 2.0 * cosim - 3.0 * cosisq);\n           f322 = -1.875 * sinim  *  (1.0 + 2.0 * cosim - 3.0 * cosisq);\n           f441 = 35.0 * sini2 * f220;\n           f442 = 39.3750 * sini2 * sini2;\n           f522 =  9.84375 * sinim * (sini2 * (1.0 - 2.0 * cosim- 5.0 * cosisq) +...\n               0.33333333 * (-2.0 + 4.0 * cosim + 6.0 * cosisq) );\n           f523 = sinim * (4.92187512 * sini2 * (-2.0 - 4.0 * cosim +...\n               10.0 * cosisq) + 6.56250012 * (1.0+2.0 * cosim - 3.0 * cosisq));\n           f542 = 29.53125 * sinim * (2.0 - 8.0 * cosim+cosisq *...\n               (-12.0 + 8.0 * cosim + 10.0 * cosisq));\n           f543 = 29.53125 * sinim * (-2.0 - 8.0 * cosim+cosisq *...\n               (12.0 + 8.0 * cosim - 10.0 * cosisq));\n           xno2  =  nm * nm;\n           ainv2 =  aonv * aonv;\n           temp1 =  3.0 * xno2 * ainv2;\n           temp  =  temp1 * root22;\n           d2201 =  temp * f220 * g201;\n           d2211 =  temp * f221 * g211;\n           temp1 =  temp1 * aonv;\n           temp  =  temp1 * root32;\n           d3210 =  temp * f321 * g310;\n           d3222 =  temp * f322 * g322;\n           temp1 =  temp1 * aonv;\n           temp  =  2.0 * temp1 * root44;\n           d4410 =  temp * f441 * g410;\n           d4422 =  temp * f442 * g422;\n           temp1 =  temp1 * aonv;\n           temp  =  temp1 * root52;\n           d5220 =  temp * f522 * g520;\n           d5232 =  temp * f523 * g532;\n           temp  =  2.0 * temp1 * root54;\n           d5421 =  temp * f542 * g521;\n           d5433 =  temp * f543 * g533;\n           xlamo =  rem(mo + nodeo + nodeo-theta - theta, twopi);\n           xfact =  mdot + dmdt + 2.0 * (nodedot + dnodt - rptim) - no;\n           em    = emo;\n           emsq  = emsqo;\n       end\n\n       % /* ---------------- synchronous resonance terms -------------- */\n       if (irez == 1)\n           g200  = 1.0 + emsq * (-2.5 + 0.8125 * emsq);\n           g310  = 1.0 + 2.0 * emsq;\n           g300  = 1.0 + emsq * (-6.0 + 6.60937 * emsq);\n           f220  = 0.75 * (1.0 + cosim) * (1.0 + cosim);\n           f311  = 0.9375 * sinim * sinim * (1.0 + 3.0 * cosim) - 0.75 * (1.0 + cosim);\n           f330  = 1.0 + cosim;\n           f330  = 1.875 * f330 * f330 * f330;\n           del1  = 3.0 * nm * nm * aonv * aonv;\n           del2  = 2.0 * del1 * f220 * g200 * q22;\n           del3  = 3.0 * del1 * f330 * g300 * q33 * aonv;\n           del1  = del1 * f311 * g310 * q31 * aonv;\n           xlamo = rem(mo + nodeo + argpo - theta, twopi);\n           xfact = mdot + xpidot - rptim + dmdt + domdt + dnodt - no;\n       end\n\n       % /* ------------ for sgp4, initialize the integrator ---------- */\n       xli   = xlamo;\n       xni   = no;\n       atime = 0.0;\n       nm    = no + dndt;\n   end\n\n\n\nsatrec.irez = irez;\nsatrec.atime = atime;\nsatrec.d2201 = d2201;\nsatrec.d2211 = d2211;\nsatrec.d3210 = d3210;\nsatrec.d3222 = d3222;\nsatrec.d4410 = d4410;\nsatrec.d4422 = d4422;\nsatrec.d5220 = d5220;\nsatrec.d5232 = d5232;\nsatrec.d5421 = d5421;\nsatrec.d5433 = d5433;\nsatrec.dedt = dedt;\nsatrec.didt = didt;\nsatrec.dmdt = dmdt;\nsatrec.dnodt = dnodt;\nsatrec.domdt = domdt;\nsatrec.del1 = del1;\nsatrec.del2 = del2;\nsatrec.del3 = del3;\nsatrec.xfact = xfact;\nsatrec.xlamo = xlamo;\nsatrec.xli = xli;\nsatrec.xni = xni;\n\n    %       [em,argpm,inclm,mm,nm,nodem,satrec.irez,satrec.atime,...\n    %           satrec.d2201,satrec.d2211,satrec.d3210,satrec.d3222,...\n     %          satrec.d4410,satrec.d4422,satrec.d5220,satrec.d5232,...\n      %         satrec.d5421,satrec.d5433,satrec.dedt,satrec.didt,...\n      %         satrec.dmdt,dndt,satrec.dnodt,satrec.domdt,satrec.del1,...\n        %       satrec.del2,satrec.del3,...\n        %       ... %ses,sghl,sghs,sgs,shl,shs,sis,sls,theta,...\n      %         satrec.xfact,satrec.xlamo,satrec.xli,satrec.xni] ...\n %= dsinit(...\n     %          cosim,emsq,satrec.argpo,s1,s2,s3,s4,s5,sinim,ss1,ss2,ss3,...\n      %         ss4,ss5,sz1,sz3,sz11,sz13,sz21,sz23,sz31,sz33,satrec.t,tc,...\n         %      satrec.gsto,satrec.mo,satrec.mdot,satrec.no,satrec.nodeo,...\n          %     satrec.nodedot,xpidot,z1,z3,z11,z13,z21,z23,z31,z33,em,...\n           %    argpm,inclm,mm,nm,nodem,satrec.ecco,eccsq);\n\n       end\n\n       % /* ----------- set variables if not deep space ----------- */\n       if (satrec.isimp ~= 1)\n           cc1sq          = satrec.cc1 * satrec.cc1;\n           satrec.d2    = 4.0 * ao * tsi * cc1sq;\n           temp           = satrec.d2 * tsi * satrec.cc1 / 3.0;\n           satrec.d3    = (17.0 * ao + sfour) * temp;\n           satrec.d4    = 0.5 * temp * ao * tsi *...\n               (221.0 * ao + 31.0 * sfour) * satrec.cc1;\n           satrec.t3cof = satrec.d2 + 2.0 * cc1sq;\n           satrec.t4cof = 0.25 * (3.0 * satrec.d3 + satrec.cc1 *...\n               (12.0 * satrec.d2 + 10.0 * cc1sq));\n           satrec.t5cof = 0.2 * (3.0 * satrec.d4 +...\n               12.0 * satrec.cc1 * satrec.d3 +...\n               6.0 * satrec.d2 * satrec.d2 +...\n               15.0 * cc1sq * (2.0 * satrec.d2 + cc1sq));\n       end\n   end % // if omeosq = 0 ...\n\n   % /* finally propogate to zero epoch to initialise all others. */\n  % if(satrec.error == 0)\n     %  [satrec, r, v] = sgp4(satrec, 0.0);\n   %end\n\n   satrec.init = 'n';"("satrec"="satrec") -> ("satrec"=→"satrec 2":T3)  [unwired: 1 in, 1 out]
